vi "Teleop - Get Datalog Names (SubVI).vi"(6 "Data Acquisition Cluster 2":T1, 10 "disabled":bool, 11 "Data Acquisition Cluster":T1) -> (2 "Data Acquisition Array out":string[][](array[string]), 3 "Array":string[](array[string]))   [LabVIEW 2019]
uses:
  Disabled/Data Acquisition Cluster.ctl
  <vilib>/Utility/Data Type/NI_Data Type.lvlib
panel:
  in  "Data Acquisition Array in":string[][](array[string])
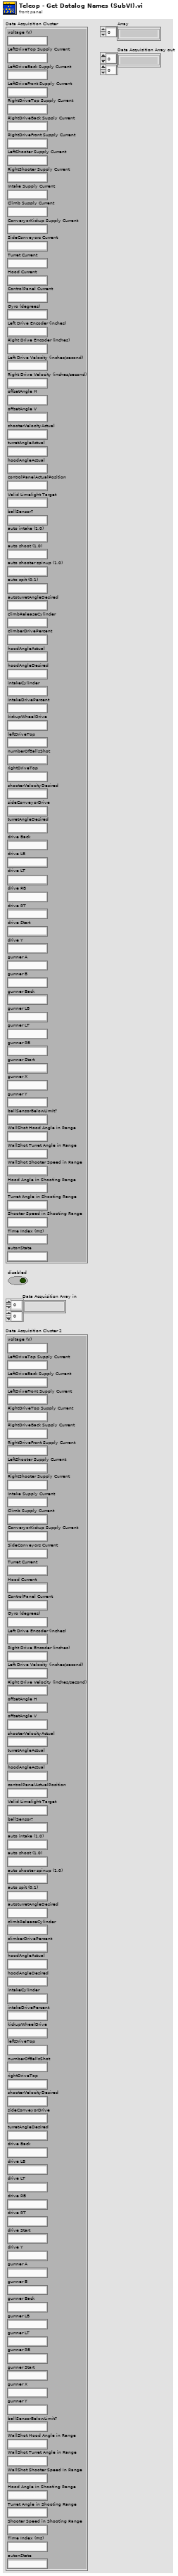
[diagram p1: front panel]
types:
  T1 = typedef "Data Acquisition Cluster.ctl" = cluster{"voltage (V)":string, "LeftDriveTop Supply Current":string, "LeftDriveBack Supply Current":string, "LeftDriveFront Supply Current":string, "RightDriveTop Supply Current":string, "RightDriveBack Supply Current":string, "RightDriveFront Supply Current":string, "LeftShooter Supply Current":string, "RightShooter Supply Current":string, "Intake Supply Current":string, "Climb Supply Current":string, "ConveryorKickup Supply Current":string, "SideConveyors Current":string, "Turret Current":string, "Hood Current":string, "ControlPanel Current":string, "Gyro (degrees)":string, "Left Drive Encoder (inches)":string, "Right Drive Encoder (inches)":string, "Left Drive Velocity (inches/second)":string, "Right Drive Velocity (inches/second)":string, "offsetAngle H":string, "offsetAngle V":string, "shooterVelocityActual":string, "turretAngleActual":string, "hoodAngleActual":string, "controlPanelActualPosition":string, "Valid Limelight Target":string, "ballSensor?":string, "auto intake (1,0)":string, "auto shoot (1,0)":string, "auto shooter spinup (1,0)":string, "auto spit (0,1)":string, "autoturretAngleDesired":string, "climbReleaseCylinder":string, "climberDrivePercent":string, "hoodAngleActual":string, "hoodAngleDesired":string, "intakeCylinder":string, "intakeDrivePercent":string, "kickupWheelDrive":string, "leftDriveTop":string, "numberOfBallsShot":string, "rightDriveTop":string, "shooterVelocityDesired ":string, "sideConveyorDrive":string, "turretAngleDesired":string, "drive Back":string, "drive LB":string, "drive LT":string, "drive RB":string, "drive RT":string, "drive Start":string, "drive Y":string, "gunner A":string, "gunner B":string, "gunner Back":string, "gunner LB":string, "gunner LT":string, "gunner RB":string, "gunner Start":string, "gunner X":string, "gunner Y":string, "ballSensorBelowLimit?":string, "WallShot Hood Angle in Range":string, "WallShot Turret Angle in Range":string, "WallShot Shooter Speed in Range":string, "Hood Angle in Shooting Range":string, "Turret Angle in Shooting Range":string, "Shooter Speed in Shooting Range":string, "Time Index (ms)":string, "autonState":string}
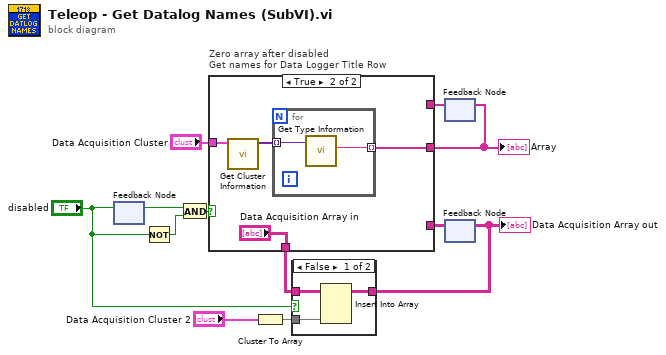
[diagram p0: block diagram]
diagram:
  n1 = feedback #1() -> (w3:bool)  [unwired: 1 in]
  n2 = feedback-in #1("disabled") -> ()
  n3 = Not(x="disabled") -> (.not. x?=w2:bool)
  n4 = And(x=w3, y=w2) -> (x .and. y?=w4:bool)
  n5 = Cluster To Array(cluster="Data Acquisition Cluster 2") -> (array=w7:string[])
  n6 = feedback #2() -> (w12:string[])  [unwired: 1 in]
  n7 = feedback #3() -> (w1:string[][])  [unwired: 1 in]
  n8 = case "Zero array after disabled\nGet names for Data Logger Title Row" shown="True" w4 {
    tunnel: w1 -> [w14 _]
    tunnel: [w14 "Data Acquisition Array in"] -> w8
    tunnel: "Data Acquisition Cluster" -> [_ w16]
    tunnel: [w13 w15] -> w11
    tunnel: w12 -> [w13 _]
    frame False {
    }
    frame True {
      n9 = call <vilib>:"Get Cluster Information.vi"("variant"=w16) -> ("cluster elements"=w17:variant[])  [unwired: 9 in, 1 out]
      n10 = for {
        tunnel: w17 -> [w20] mode=indexing
        tunnel: [w19] -> w15 mode=indexing
        n11 = call <vilib>:"Get Type Information.vi"("variant"=w20) -> ("name"=w19:string)  [unwired: 6 in, 4 out]
      }
    }
  }
  "Array" <- w11
  n12 = case shown="False" "disabled" {
    tunnel: w7 -> [w23 _]
    tunnel: [w22 w24] -> w9
    tunnel: w8 -> [w21 w24]
    frame False {
      n13 = Insert Into Array(array=w21, new element=w23) -> (w22:string[][])  [unwired: 2 in]
    }
    frame True {
    }
  }
  "Data Acquisition Array out" <- w9
  n14 = feedback-in #2(w11) -> ()
  n15 = feedback-in #3(w9) -> ()
